vi "getState.vi"(8 "error in (no error)":errorcluster, 11 "OfflineState in":refnum<class "OfflineState.lvclass">) -> (0 "error out":errorcluster, 2 "DeviceStatus":T1, 3 "OfflineState out":refnum<class "OfflineState.lvclass">)   [LabVIEW 2016, in "OfflineState.lvclass"]
uses:
  OfflineState.lvclass
  Typedefs/DeviceStatus.ctl
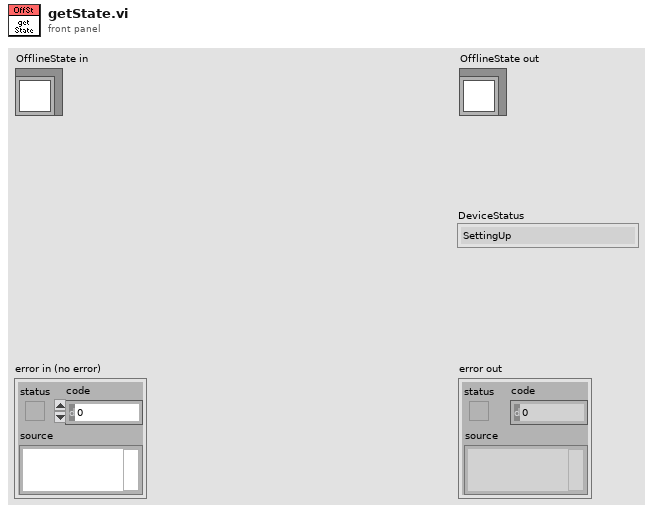
[diagram p1: front panel]
types:
  T1 = typedef "DeviceStatus.ctl" = enum16{"SettingUp", "Ready", "Offline", "Fault"}
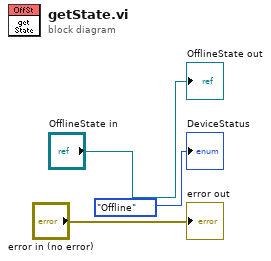
[diagram p0: block diagram]
diagram:
  "error out" <- "error in (no error)"
  "OfflineState out" <- "OfflineState in"
  "DeviceStatus" <- DeviceStatus."Offline" ("DeviceStatus")
